vi "Config - ReadFile.vi"(8 "Fehler (Eingang, kein Fehler)":errorcluster, 10 "DestinationFullFileName":string, 11 "SourceFileName":string) -> (0 "Fehler (Ausgang)":errorcluster)   [LabVIEW 2016]
uses:
  eGateUtility.dll
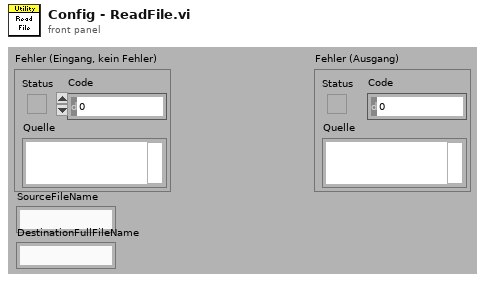
[diagram p1: front panel]
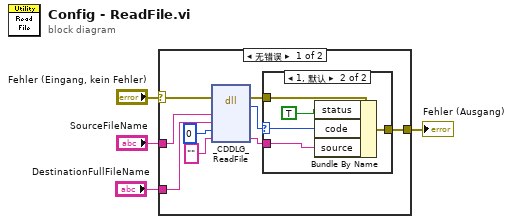
[diagram p0: block diagram]
diagram:
  n1 = case shown="无错误" "Fehler (Eingang, kein Fehler)" {
    selector: "Fehler (Eingang, kein Fehler)" -> [w11 w20]
    tunnel: [w9 w20] -> w3
    tunnel: "SourceFileName" -> [w6 _]
    tunnel: "DestinationFullFileName" -> [w5 _]
    frame No Error {
      n2 = dll-call lib="eGateUtility.dll" fn="_CDDLG_ReadFile"(error in=w11, "SourceFileName"=w6, "DestinationFullFileName"=w5, "AppendToExisting"=0, "ErrorString"="") -> (error out=w10:errorcluster, "Rückgabetyp"=w7:i32, "ErrorString"=w8:string)  [unwired: 5 in, 1 out]
      n3 = case shown="1, 默认" w7 {
        selector: w7 -> [_ w16]
        tunnel: w10 -> [w14 w19]
        tunnel: [w14 w18] -> w9
        tunnel: w8 -> [_ w17]
        frame 0 {
        }
        frame 1, Default {
          n4 = Bundle By Name(cluster=w19, "status"=TRUE, "code"=w16, "source"=w17) -> (w18:errorcluster)
        }
      }
    }
    frame Error {
    }
  }
  "Fehler (Ausgang)" <- w3
